vi "ISO_Week_Number.vi"(0 "seconds (now)":dbl format="%<%X\n%x>T") -> (1 "ISO date":T1, 2 "ISO week":i32)   [LabVIEW 2013]
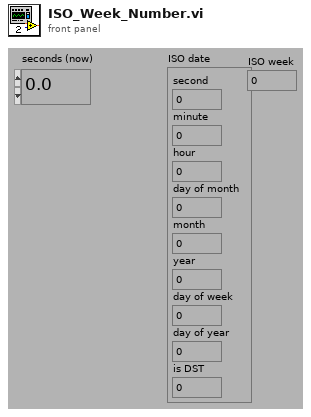
[diagram p1: front panel]
types:
  T1 = cluster{"second":i32, "minute":i32, "hour":i32, "day of month":i32, "month":i32, "year":i32, "day of week":i32, "day of year":i32, "is DST":i32}
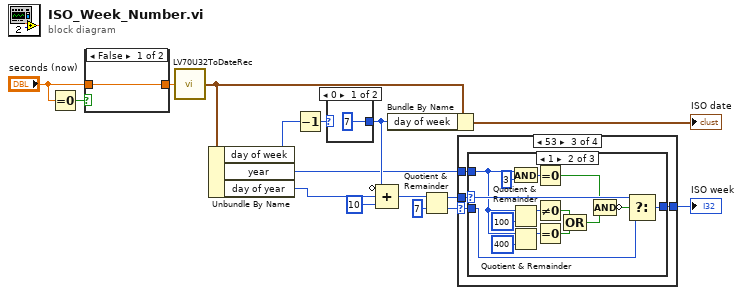
[diagram p0: block diagram]
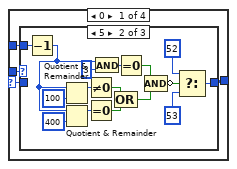
[diagram p2: hidden frame]
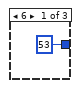
[diagram p3: hidden frame]
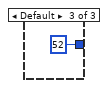
[diagram p4: hidden frame]
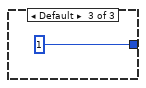
[diagram p7: hidden frame]
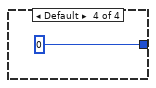
[diagram p8: hidden frame]
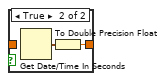
[diagram p10: hidden frame]
diagram:
  n1 = Equal To 0?(x="seconds (now)") -> (x = 0?=w13:bool)
  n2 = case shown="False" w13 {
    tunnel: [w17 w18] -> w14
    tunnel: "seconds (now)" -> [w17 _]
    frame False {
    }
    frame True {
      n3 = Get Date/Time In Seconds() -> (seconds since 1Jan1904=w19:timestamp)
      n4 = To Double Precision Float(number=w19) -> (double precision float=w18:dbl)
    }
  }
  n5 = call <vilib>:"LV70U32ToDateRec.vi"("Time"=w14) -> ("date time rec"=w16:T1)
  n6 = Unbundle By Name(w16) -> ("day of week"=w7:i32, "year"=w2:i32, "day of year"=w1:i32)
  n7 = Decrement(x=w7) -> (x-1=w8:i32)
  n8 = case shown="0" w8 {
    selector: w8 -> [_ w21]
    tunnel: [7 ("day of week") w21] -> w6
    frame 0 {
    }
    frame Default {
    }
  }
  n9 = Compound Arithmetic op=ADD(invert w6, w1, 10 ("Input")) -> (w10:i32)
  n10 = Bundle By Name(cluster=w16, "day of week"=w6) -> (→"ISO date":T1)
  n11 = Quotient & Remainder(x=w10, y=7) -> (x-y*floor(x/y)=w4:i32, floor(x/y)=w5:i32)
  n12 = case shown="53" w5 {
    selector: w5 -> [w25 w44 w46 _]
    tunnel: [w23 w44 w47 0] -> w3
    tunnel: w4 -> [w24 _ w48 _]
    tunnel: w2 -> [w22 _ w45 _]
    frame 0 {
      n13 = case shown="5" w24 {
        tunnel: [53 w42 52 ("t")] -> w23
        tunnel: w25 -> [_ _ _]
        tunnel: w22 -> [_ w27 _]
        frame 6 {
        }
        frame 5 {
          n14 = Decrement(x=w27) -> (x-1=w30:i32)
          n15 = Quotient & Remainder(x=w30, y=100) -> (x-y*floor(x/y)=w39:i32)  [unwired: 1 out]
          n16 = Quotient & Remainder(x=w30, y=400) -> (x-y*floor(x/y)=w40:i32)  [unwired: 1 out]
          n17 = Not Equal To 0?(x=w39) -> (x != 0?=w34:bool)
          n18 = Equal To 0?(x=w40) -> (x = 0?=w33:bool)
          n19 = And(x=w30, y=3) -> (x .and. y?=w38:i32)
          n20 = Compound Arithmetic op=OR(w34, w33) -> (w32:bool)
          n21 = Equal To 0?(x=w38) -> (x = 0?=w41:bool)
          n22 = Compound Arithmetic op=AND(w41, w32) -> (invert w35:bool)
          n23 = Select(t=52, s=w35, f=53 ("t")) -> (s? t:f=w42:i32)
        }
        frame Default {
        }
      }
    }
    frame 1..52 {
    }
    frame 53 {
      n24 = case shown="1" w48 {
        selector: w48 -> [_ w63 _]
        tunnel: [w49 w64 1] -> w47
        tunnel: w46 -> [w49 w62 _]
        tunnel: w45 -> [_ w50 _]
        frame 0 {
        }
        frame 1 {
          n25 = And(x=w50, y=3) -> (x .and. y?=w58:i32)
          n26 = Quotient & Remainder(x=w50, y=100) -> (x-y*floor(x/y)=w59:i32)  [unwired: 1 out]
          n27 = Quotient & Remainder(x=w50, y=400) -> (x-y*floor(x/y)=w60:i32)  [unwired: 1 out]
          n28 = Equal To 0?(x=w58) -> (x = 0?=w61:bool)
          n29 = Not Equal To 0?(x=w59) -> (x != 0?=w53:bool)
          n30 = Equal To 0?(x=w60) -> (x = 0?=w52:bool)
          n31 = Compound Arithmetic op=OR(w53, w52) -> (w51:bool)
          n32 = Compound Arithmetic op=AND(w61, w51) -> (invert w54:bool)
          n33 = Select(t=w63, s=w54, f=w62) -> (s? t:f=w64:i32)
        }
        frame Default {
        }
      }
    }
    frame Default {
    }
  }
  "ISO week" <- w3
